vi "Ej_8_Concatenar_String.vi"() -> ()   [LabVIEW 2021]
panel:
  out "output 3":dbl
  out "after substring 3":string
  out "offset past match 2":i32
  out "output 2":dbl
  out "after substring 2":string
  out "output 1":dbl
  out "after substring":string
  out "match substring":string
  out "before substring":string
  in  "Medición":dbl
  in  "Unidades":string="Volts"
  out "Longitud":i32
  in  "Encabezado":string="El Valor Del Voltaje Es:"
  out "concatenated string":string
  out "offset past match":i32
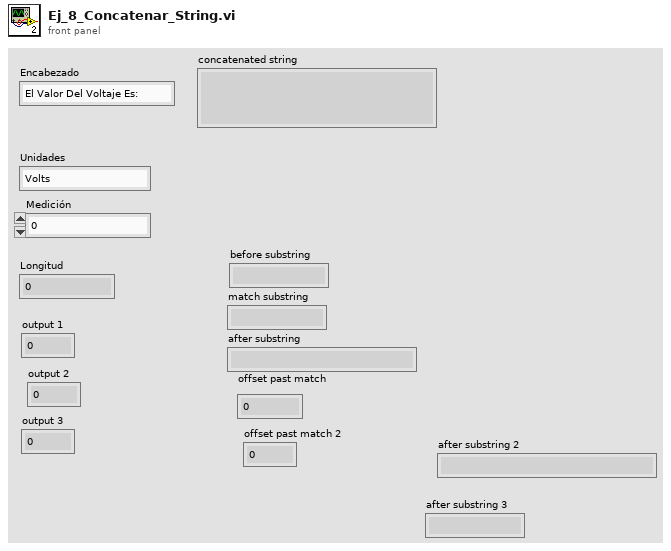
[diagram p1: front panel]
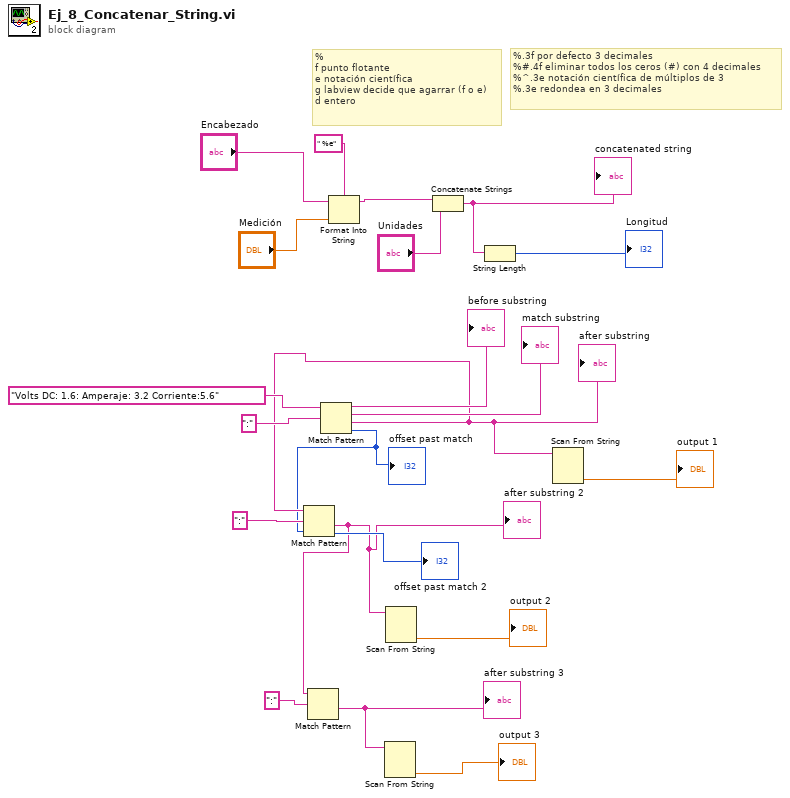
[diagram p0: block diagram]
diagram:
  # "%.3f por defecto 3 decimales\n%#.4f eliminar todos los ceros (#) con 4 decimales \n%^.3e notación científica de múltiplos de 3\n%.3e redondea en 3 decimales"
  # "%\nf punto flotante\ne notación científica\ng labview decide que agarrar (f o e)\nd entero"
  n1 = Match Pattern(string="Volts DC: 1.6: Amperaje: 3.2 Corriente:5.6", regular expression=":") -> (before substring=→"before substring":string, match substring=→"match substring":string, after substring=w7:string, offset past match=w6:i32)  [unwired: 1 in]
  "offset past match" <- w6
  "after substring" <- w7
  n2 = Match Pattern(string=w7, regular expression=":", offset (0)=w6) -> (after substring=w4:string, offset past match=→"offset past match 2":i32)  [unwired: 2 out]
  "after substring 2" <- w4
  n3 = Match Pattern(string=w4, regular expression=":") -> (after substring=w2:string)  [unwired: 1 in, 3 out]
  "after substring 3" <- w2
  n4 = Format Into String "Format Into String"(format string=" %e", initial string="Encabezado", "Medición") -> (resulting string=w18:string)  [unwired: 1 in, 1 out]
  n5 = Scan From String "Scan From String"(input string=w2) -> (output 1=→"output 3":dbl)  [unwired: 4 in, 3 out]
  n6 = Scan From String "Scan From String"(input string=w4) -> (output 1=→"output 2":dbl)  [unwired: 4 in, 3 out]
  n7 = Concatenate Strings "Concatenate Strings"(w18, "Unidades") -> (w16:string)
  "concatenated string" <- w16
  n8 = String Length(string=w16) -> (length=→"Longitud":i32)
  n9 = Scan From String "Scan From String"(input string=w7) -> (output 1=→"output 1":dbl)  [unwired: 4 in, 3 out]
